vi "Set Waveform Vertical Offset.vi"(8 "error in (no error)":errorcluster, 9 "Offset Divisions":dbl, 10 "Analog Channels":T1, 11 "MSOX6004 in":refnum<class "MSOX6004.lvclass">) -> (0 "error out":errorcluster, 3 "MSOX6004 out":refnum<class "MSOX6004.lvclass">)   [LabVIEW 2018, in "MSOX6004.lvlib" / "MSOX6004.lvclass"]
doc: "This Override is used to change the vertical placement individual waveforms."
uses:
  MSOX6004.lvclass
  PPLs/Oscilloscope/Parent/Oscilloscope.lvlibp/Custom Controls/Analog Channels.ctl
  MSOX6004.lvclass/MSOX6004.ctl
  <instrlib>/Keysight InfiniiVision/Keysight InfiniiVision.lvlib
  PPLs/Oscilloscope/Parent/Oscilloscope.lvlibp
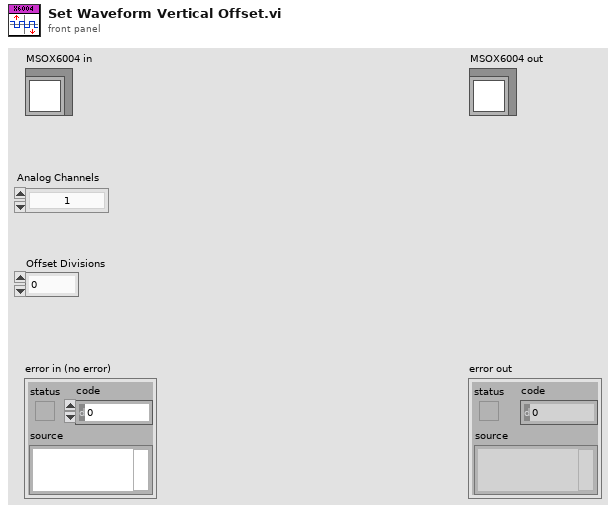
[diagram p1: front panel]
types:
  T1 = typedef "Oscilloscope.lvlibp/Analog Channels.ctl" = enum16{"1", "2", "3", "4", "5", "6", "7", "8", "9", "10", "11", "12", "13", "14", "15", "16"}
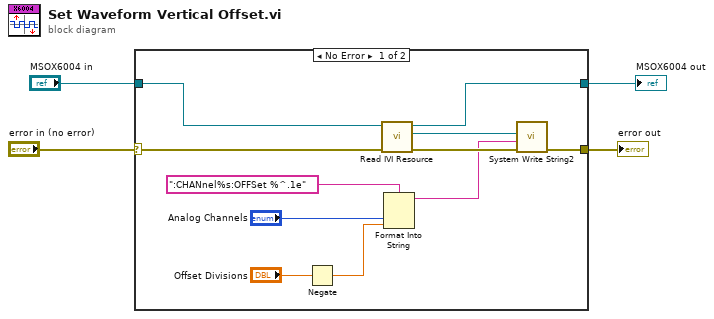
[diagram p0: block diagram]
diagram:
  n1 = case shown="No Error" "error in (no error)" {
    selector: "error in (no error)" -> [w13 w16]
    tunnel: "MSOX6004 in" -> [w12 w17]
    tunnel: [w11 w17] -> w2
    tunnel: [w7 w16] -> w1
    frame No Error {
      n2 = Negate(x="Offset Divisions") -> (-x=w5:dbl)
      n3 = call "Read IVI Resource.vi"("error in (no error)"=w13, "MSOX6004 in"=w12) -> ("error out"=w9:errorcluster, "IVI Resource"=w10:refnum<k15>, "MSOX6004 out"=w11:refnum<class "MSOX6004.lvclass">)  [unwired: 7 in]
      n4 = Format Into String(format string=":CHANnel%s:OFFSet %^.1e" ("channel name"), "Analog Channels", w5) -> (resulting string=w8:string)  [unwired: 2 in, 1 out]
      n5 = call <instrlib>:"System Write String2.vi"("error in (no error)"=w9, "Data"=w8, "instrument handle"=w10) -> ("error out"=w7:errorcluster)  [unwired: 7 in, 1 out]
    }
    frame Error {
    }
  }
  "error out" <- w1
  "MSOX6004 out" <- w2
